vi "Project Items - Keep Virtual Folders.vi"(8 "Error In":errorcluster, 11 "Project Items":refnum<vi>[](array[refnum])) -> (0 "Error Out":errorcluster, 3 "Project Items (Folders)":refnum<vi>[](array[refnum]))   [LabVIEW 2022 SP3]
doc: "<add documentation here>"
panel:
  # "Development\nControls or indicators that are useful for development or testing, but which are not outputs of the VI."
  # "Input\nInputs to the VI"
  # "Output\nOutputs of the VI"
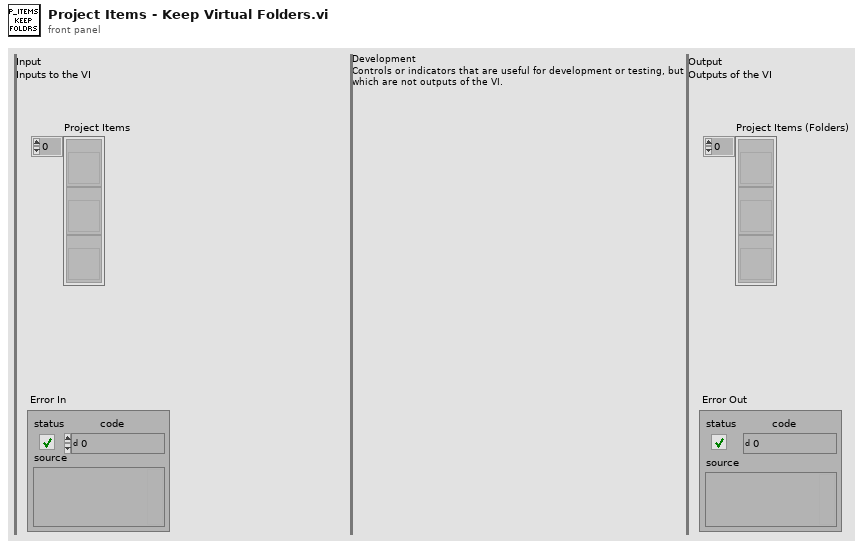
[diagram p1: front panel]
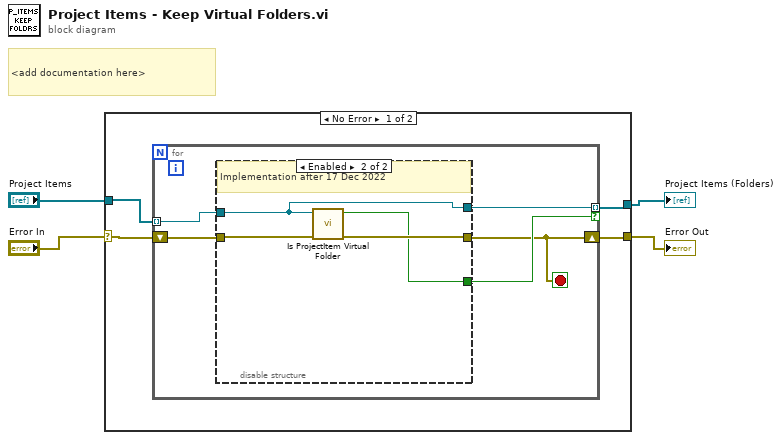
[diagram p0: block diagram]
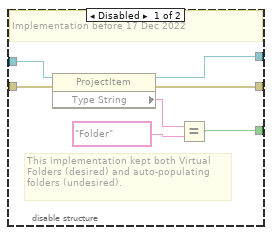
[diagram p2: hidden frame]
diagram:
  # "<add documentation here>"
  n1 = case shown="No Error" "Error In" {
    selector: "Error In" -> [w8 w25]
    tunnel: [w6 w25] -> w3
    tunnel: "Project Items" -> [w7 _]
    tunnel: [w5 _] -> w1
    frame No Error {
      n2 = for {
        tunnel: w7 -> [w13] mode=indexing
        shift-right: [w9] -> w6
        shift-left: w8 -> [w12]
        tunnel: [w11] -> w5 mode=indexing if=w10
        stop <- w9 stop-if-true
        n3 = disable-structure shown="Enabled" {
          disable-tunnel: w13 -> [w20 w21]
          disable-tunnel: w12 -> [w19 w24]
          disable-tunnel: [w16 w21] -> w11
          disable-tunnel: [w15 w22] -> w10
          disable-tunnel: [w14 w23] -> w9
          frame Disabled {
            # "This implementation kept both Virtual Folders (desired) and auto-populating folders (undesired)."
            # "Implementation before 17 Dec 2022"
            n4 = property class="ProjectItem"(reference=w20, error in=w19) -> (reference out=w16:refnum<vi>, error out=w14:errorcluster, "Type String"=w18:string)
            n5 = Equal?(x=w18, y="Folder") -> (x = y?=w15:bool)
          }
          frame Enabled {
            # "Implementation after 17 Dec 2022"
            n6 = call "Is ProjectItem Virtual Folder.vi"("Error In"=w24, "ProjectItem Refnum"=w21) -> ("Error Out"=w23:errorcluster, "Is Virtual Folder?"=w22:bool)  [unwired: 8 in]
          }
        }
      }
    }
    frame Error {
    }
  }
  "Error Out" <- w3
  "Project Items (Folders)" <- w1
